vi "Load 1PLOT.vi"(8 "error in (no error)":errorcluster, 10 "Filepath":path, 11 "BlueSerializer in":refnum<class "BlueSerializer.lvclass">) -> (0 "error out":errorcluster, 2 "SerializableData.Plot config":T1={"plots"=[], "X-axis"={"Name Label.Text"="", "Style"=0, "Tick Colors:Minor Tick Color"=0, "Tick Colors:Tick Color"=0, "Marker Colors:Text Color"=0, "Grid Colors:Major Color"=0, "Grid Colors:Minor Color"=0, "Mapping Mode"=0, "Flipped"=FALSE, "Name Label.Visible"=FALSE, "Name Label.Text Colors:Text Color"=0, "Scale Fit"=0, "Editable"=FALSE, "Range:Maximum"=0.0, "Range:Minimum"=0.0, "Offset and Multiplier:Multiplier"=0.0, "Offset and Multiplier:Offset"=0.0, "Name Label.Font:Size"=0, "Marker.Font:Size"=0, "Uniform Marker Spacing?"=TRUE, "Format String"=""}, "Y-axes"=[], "General"={"Title"="", "Time to Plot"=1800.0, "Title.Visible"=FALSE, "Sidebar.Visible"=FALSE, "Plot Area:Colors:BG Color"=0}} {"General"."Time to Plot" format="%<%M:%S>t"}, 3 "BlueSerializer out":refnum<class "BlueSerializer.lvclass">)   [LabVIEW 2021, in "BluePlot.lvlib" / "BlueSinglePlotConfig.lvclass"]
uses:
  BlueSinglePlotConfig.lvclass
  BlueSinglePlotConfig.lvclass/BlueSinglePlotConfig.ctl
  46e0e9db-e893-4c3f-8c80-cb7d509b4b92.vi
  <userlib>/Blue Origin/BlueSerialization/BlueSerializer/BlueSerializer.lvclass
  TypeDefs/plot attributes V2.ctl
  BluePlot.lvlib
  TypeDefs/plot properties V2.ctl
  TypeDefs/Plot scale axis properties.ctl
  TypeDefs/Plot general properties.ctl
  TypeDefs/plot load data V2.ctl
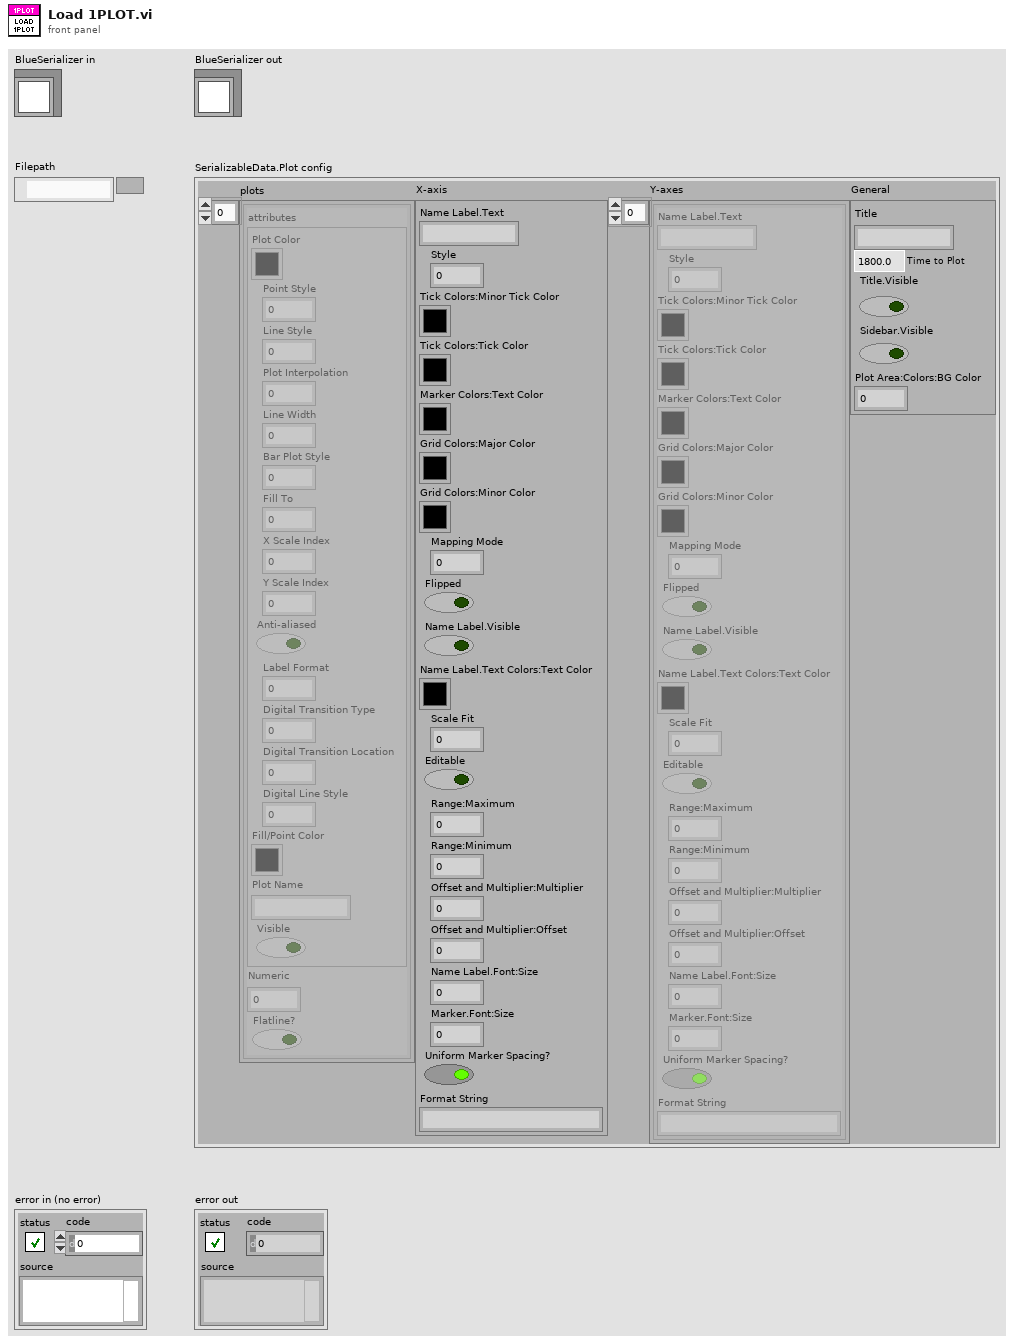
[diagram p1: front panel]
types:
  T1 = typedef "BluePlot.lvlib/plot load data V2.ctl" = cluster{"plots":T2[], "X-axis":T4, "Y-axes":T4[], "General":T5}
  T2 = typedef "BluePlot.lvlib/plot properties V2.ctl" = cluster{"attributes":T3, "Numeric":dbl, "Flatline?":bool}
  T3 = typedef "BluePlot.lvlib/plot attributes V2.ctl" = cluster{"Plot Color":u32, "Point Style":u8, "Line Style":u8, "Plot Interpolation":u8, "Line Width":u8, "Bar Plot Style":u8, "Fill To":i16, "X Scale Index":u32, "Y Scale Index":u32, "Anti-aliased":bool, "Label Format":u8, "Digital Transition Type":u8, "Digital Transition Location":u8, "Digital Line Style":u8, "Fill/Point Color":u32, "Plot Name":string, "Visible":bool}
  T4 = typedef "BluePlot.lvlib/Plot scale axis properties.ctl" = cluster{"Name Label.Text":string, "Style":u8, "Tick Colors:Minor Tick Color":u32, "Tick Colors:Tick Color":u32, "Marker Colors:Text Color":u32, "Grid Colors:Major Color":u32, "Grid Colors:Minor Color":u32, "Mapping Mode":u8, "Flipped":bool, "Name Label.Visible":bool, "Name Label.Text Colors:Text Color":u32, "Scale Fit":u8, "Editable":bool, "Range:Maximum":dbl, "Range:Minimum":dbl, "Offset and Multiplier:Multiplier":dbl, "Offset and Multiplier:Offset":dbl, "Name Label.Font:Size":u32, "Marker.Font:Size":u32, "Uniform Marker Spacing?":bool, "Format String":string}
  T5 = typedef "BluePlot.lvlib/Plot general properties.ctl" = cluster{"Title":string, "Time to Plot":dbl, "Title.Visible":bool, "Sidebar.Visible":bool, "Plot Area:Colors:BG Color":u32}
  T6 = enum16{"open", "replace", "create", "open or create", "replace or create", "replace or create with confirmation"}
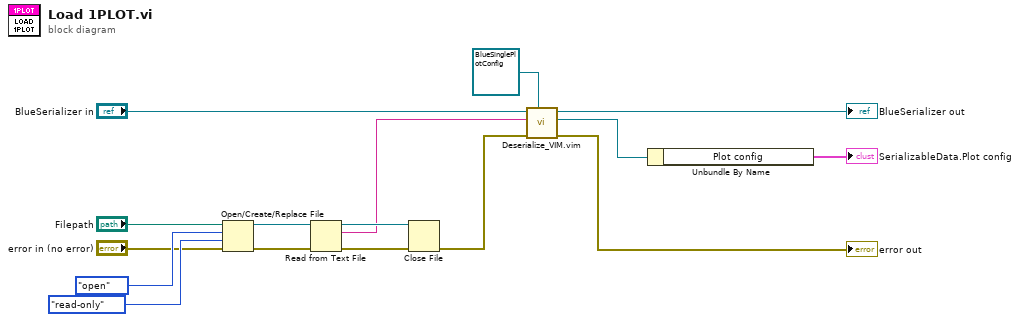
[diagram p0: block diagram]
diagram:
  n1 = Open/Create/Replace File(file path (use dialog)="Filepath", error in="error in (no error)", operation (0:open)=T6."open", access (0:read/write)=enum16{"read/write", "read-only", "write-only"}."read-only") -> (refnum out=w13:refnum<file>, error out=w11:errorcluster)  [unwired: 2 in, 1 out]
  n2 = Read from Text File(file (use dialog)=w13, error in=w11) -> (refnum out=w12:refnum<file>, text=w8:string, error out=w10:errorcluster)  [unwired: 2 in, 1 out]
  n3 = Close File(refnum=w12, error in=w10) -> (error out=w6:errorcluster)  [unwired: 1 out]
  n4 = call "Deserialize_VIM.vim"("Anything"=refnum<class "BlueSinglePlotConfig.lvclass"> refnum ("BlueSinglePlotConfig"), "error in (no error)"=w6, "Serialized Text"=w8, "BlueSerializer in"="BlueSerializer in") -> ("error out"=→"error out":errorcluster, "Data out"=w2:refnum<class "BlueSinglePlotConfig.lvclass">, "BlueSerializer out"=→"BlueSerializer out":refnum<class "BlueSerializer.lvclass">)  [unwired: 5 in]
  n5 = Unbundle By Name(w2) -> ("Plot config"=→"SerializableData.Plot config":T1)
